vi "Spindexer_Execute.vi"() -> ()   [LabVIEW 2019]
uses:
  Globals/Spindexer_Globals.vi
  <vilib>/Rock Robotics/WPI/ThirdParty/Phoenix-LabVIEW/Motor Controller/Controls/CTRE_Phoenix_MotorControl_ControlMode.ctl
panel:
  in  "Speed control velocity":dbl
  in  "Sensor 5 input":dbl
  in  "Sensor 4 input":dbl
  in  "Sensor 3 input":dbl
  in  "Sensor 2 input":dbl
  in  "Sensor 1 input":dbl
  in  "offset 5":dbl
  in  "Sensor Tolerance 5":dbl
  in  "offset 4":dbl
  in  "Sensor Tolerance 4":dbl
  in  "offset 3":dbl
  in  "Sensor Tolerance 3":dbl
  in  "offset 2":dbl
  in  "Sensor Tolerance 2":dbl
  in  "offset":dbl
  in  "Sensor Tolerance":dbl
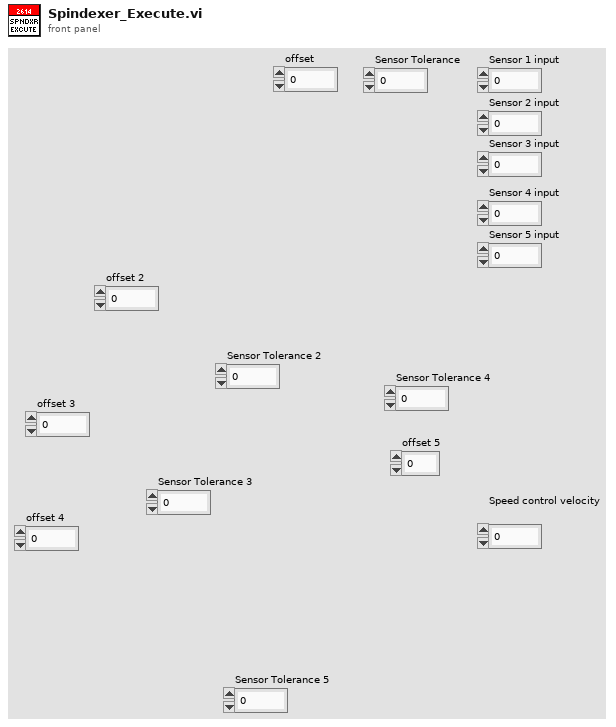
[diagram p1: front panel]
types:
  T1 = typedef "Spindexer_Cluster.ctl" = cluster{"Throttle":dbl, "Fire?":bool, "Intake recently moved?":bool, "Mode":T2, "Sensor in position? ":bool}
  T2 = typedef "Spindexer_mode.ctl" = enum16{"No-Op", "Sensing", "Intaking", "Firing(Speed Control)", "Manual"}
  T3 = typedef "CTRE_Phoenix_MotorControl_ControlMode.ctl" = u16
  T4 = typedef "WPI_MotorControlDeviceRef.ctl" = cluster{"DeviceStatus":errorcluster, "Type":T5, "PWM":cluster{"PWM Channel":T6, "DeadBand":T7}, "CAN":cluster{"Device Number":u8, "SetOutput VI Ref":variant, "GetOutput VI Ref":variant, "Enable VI Ref":variant, "Disable VI Ref":variant, "Data":variant}, "Invert":bool, "DIO PWM":cluster{"PWM \"Enable\" Channel":T6, "DIOChannel":T8, "PWM Rate":dbl}}
  T5 = typedef "WPI_MotorControlType.ctl" = enum16{"PWM", "CAN", "DIO PWM"}
  T6 = typedef "FPGA_DIOPWMChannel.ctl" = enum8{"PWM 0", "PWM 1", "PWM 2", "PWM 3", "PWM 4", "PWM 5", "PWM 6", "PWM 7", "PWM 8", "PWM 9", "PWM MXP 0", "PWM MXP 1", "PWM MXP 2", "PWM MXP 3", "PWM MXP 4", "PWM MXP 5", "PWM MXP 6", "PWM MXP 7", "PWM MXP 8", "PWM MXP 9", "Invalid"}
  T7 = typedef "WPI_PWMDeadband.ctl" = cluster{"Name":string, "maxPositivePwm":i32, "minPositivePwm":i32, "centerPwm":i32, "maxNegativePwm":i32, "minNegativePwm":i32, "angularRange":u16}
  T8 = typedef "FPGA_DIOChannel.ctl" = enum8{"DIO 0", "DIO 1", "DIO 2", "DIO 3", "DIO 4", "DIO 5", "DIO 6", "DIO 7", "DIO 8", "DIO 9", "DIO MXP 0", "DIO MXP 1", "DIO MXP 2", "DIO MXP 3", "DIO MXP 4", "DIO MXP 5", "DIO MXP 6", "DIO MXP 7", "DIO MXP 8", "DIO MXP 9", "DIO MXP 10", "DIO MXP 11", "DIO MXP 12", "DIO MXP 13", "DIO MXP 14", "DIO MXP 15", "SPI Port CS1", "SPI Port CS2", "SPI Port CS3", "SPI Port MISO", "SPI Port MOSI", "Invalid"}
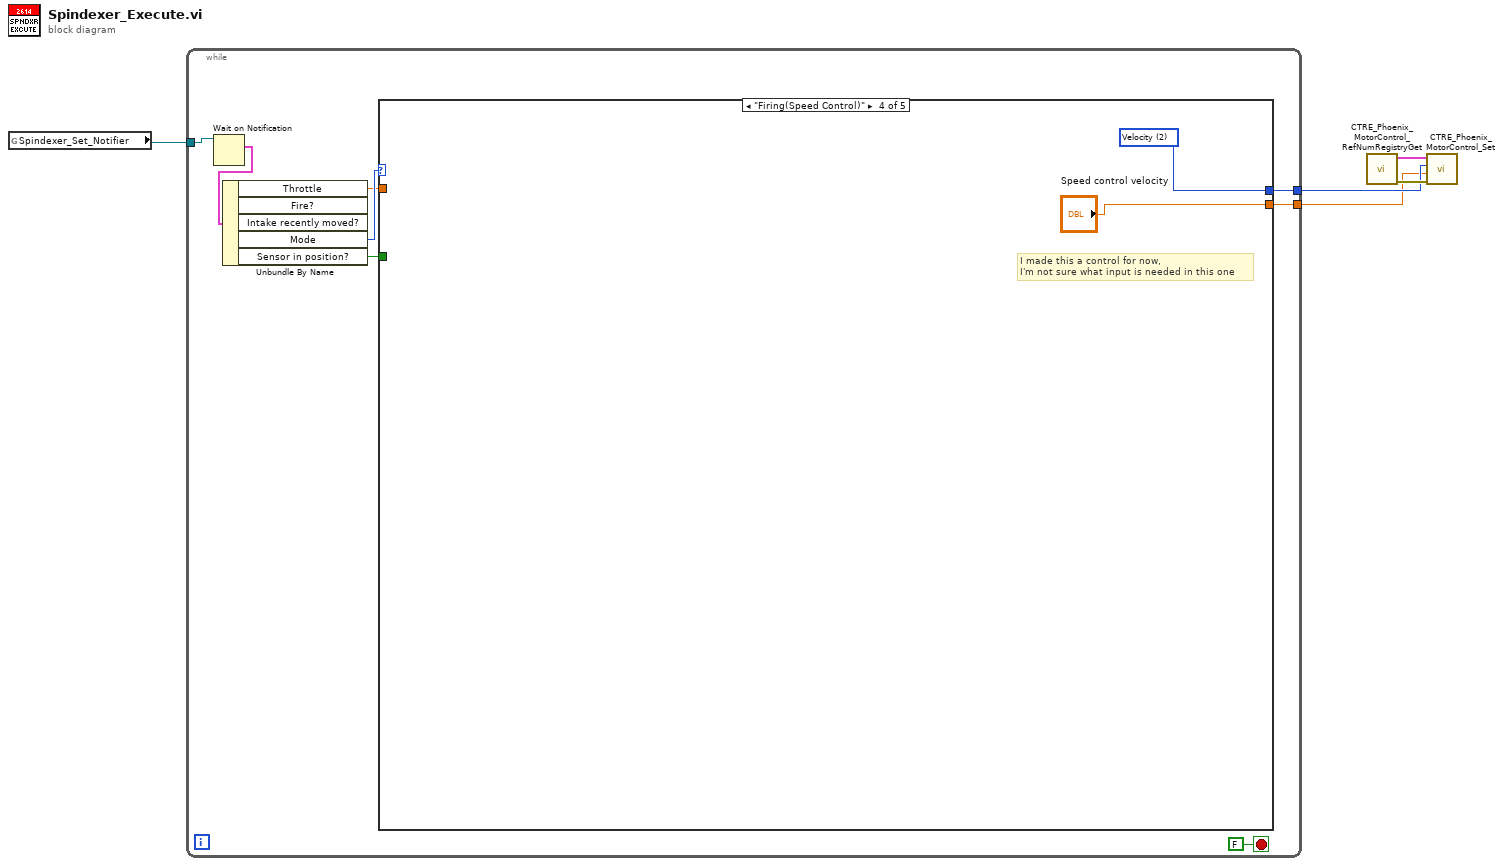
[diagram p0: block diagram]
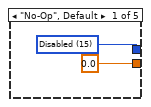
[diagram p2: hidden frame]
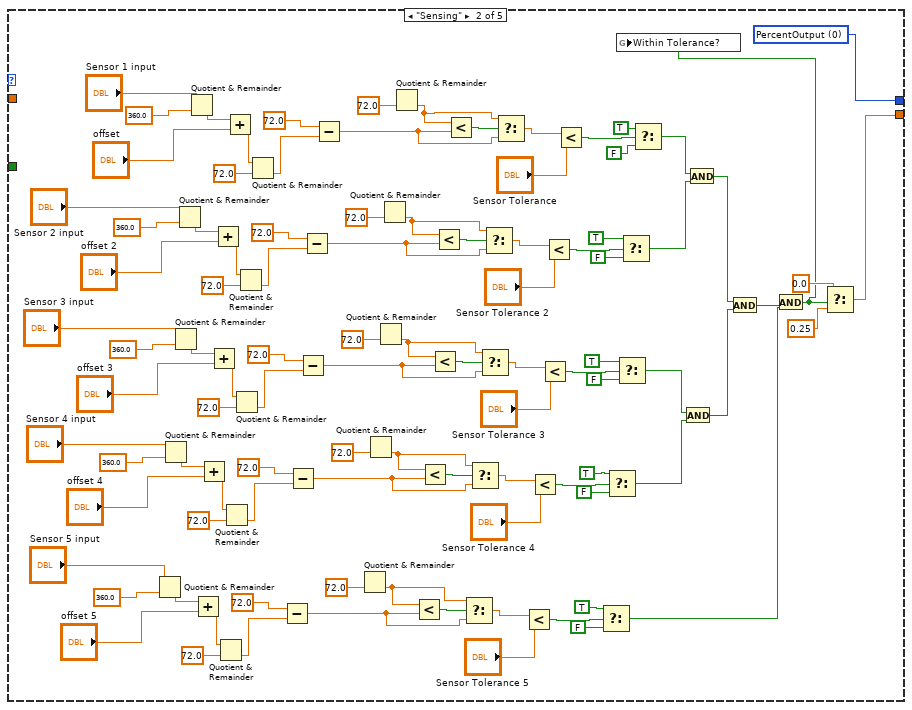
[diagram p3: hidden frame]
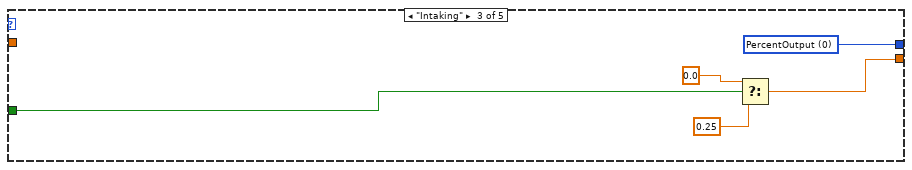
[diagram p4: hidden frame]
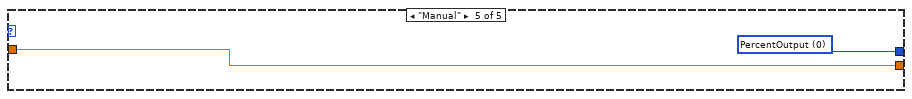
[diagram p5: hidden frame]
diagram:
  n1 = global read "Spindexer_Globals.vi" "Spindexer_Set_Notifier"() -> (w5:refnum<notifier>)
  n2 = while {
    tunnel: w5 -> [w12]
    tunnel: [w9] -> w2
    tunnel: [w7] -> w1
    stop <- FALSE stop-if-true
    n3 = Wait on Notification(notifier=w12) -> (notification=w11:T1)  [unwired: 3 in, 3 out]
    n4 = Unbundle By Name(w11) -> ("Throttle"=w8:dbl, "Mode"=w10:T2, "Sensor in position?"=w6:bool)  [unwired: 2 out]
    n5 = case shown="\"Firing(Speed Control)\"" w10 {
      tunnel: [w14 w113 w118 w120 w121] -> w9
      tunnel: w8 -> [_ _ _ _ w122]
      tunnel: [0.0 ("Throttle") w17 w114 "Speed control velocity" w122] -> w7
      tunnel: w6 -> [_ _ w117 _ _]
      frame "No-Op", Default {
        w14 = T3 15 items=["PercentOutput"=0, "Position"=1, "Velocity"=2, "Current"=3, "Follower"=5, "MotionProfile"=6, "MotionMagic"=7, "MotionProfileArc"=10, "Disabled"=15] ("Control Mode")
      }
      frame "Sensing" {
        w113 = T3 0 items=["PercentOutput"=0, "Position"=1, "Velocity"=2, "Current"=3, "Follower"=5, "MotionProfile"=6, "MotionMagic"=7, "MotionProfileArc"=10, "Disabled"=15] ("Control Mode")
        n6 = Quotient & Remainder(x="Sensor 5 input", y=360.0) -> (floor(x/y)=w53:dbl)  [unwired: 1 out]
        n7 = Quotient & Remainder(x="Sensor 4 input", y=360.0) -> (floor(x/y)=w65:dbl)  [unwired: 1 out]
        n8 = Quotient & Remainder(x="Sensor 3 input", y=360.0) -> (floor(x/y)=w77:dbl)  [unwired: 1 out]
        n9 = Quotient & Remainder(x="Sensor 2 input", y=360.0) -> (floor(x/y)=w89:dbl)  [unwired: 1 out]
        n10 = Quotient & Remainder(x="Sensor 1 input", y=360.0) -> (floor(x/y)=w101:dbl)  [unwired: 1 out]
        n11 = Add(x=w53, y="offset 5") -> (x+y=w52:dbl)
        n12 = Add(x=w65, y="offset 4") -> (x+y=w64:dbl)
        n13 = Add(x=w77, y="offset 3") -> (x+y=w76:dbl)
        n14 = Add(x=w89, y="offset 2") -> (x+y=w88:dbl)
        n15 = Quotient & Remainder(x=w52, y=72.0) -> (floor(x/y)=w61:dbl)  [unwired: 1 out]
        n16 = Quotient & Remainder(x=w64, y=72.0) -> (floor(x/y)=w73:dbl)  [unwired: 1 out]
        n17 = Add(x=w101, y="offset") -> (x+y=w100:dbl)
        n18 = Quotient & Remainder(x=w76, y=72.0) -> (floor(x/y)=w85:dbl)  [unwired: 1 out]
        n19 = Quotient & Remainder(x=w88, y=72.0) -> (floor(x/y)=w97:dbl)  [unwired: 1 out]
        n20 = Quotient & Remainder(x=w100, y=72.0) -> (floor(x/y)=w111:dbl)  [unwired: 1 out]
        n21 = Subtract(x=72.0, y=w61) -> (x-y=w58:dbl)
        n22 = Subtract(x=72.0, y=w73) -> (x-y=w70:dbl)
        n23 = Subtract(x=72.0, y=w85) -> (x-y=w82:dbl)
        n24 = Subtract(x=72.0, y=w97) -> (x-y=w94:dbl)
        n25 = Subtract(x=72.0, y=w111) -> (x-y=w106:dbl)
        n26 = Quotient & Remainder(y=72.0) -> (floor(x/y)=w50:dbl)  [unwired: 1 in, 1 out]
        n27 = Quotient & Remainder(y=72.0) -> (floor(x/y)=w45:dbl)  [unwired: 1 in, 1 out]
        n28 = Quotient & Remainder(y=72.0) -> (floor(x/y)=w44:dbl)  [unwired: 1 in, 1 out]
        n29 = Quotient & Remainder(y=72.0) -> (floor(x/y)=w43:dbl)  [unwired: 1 in, 1 out]
        n30 = Quotient & Remainder(y=72.0) -> (floor(x/y)=w107:dbl)  [unwired: 1 in, 1 out]
        n31 = Less?(x=w50, y=w58) -> (x < y?=w59:bool)
        n32 = Less?(x=w45, y=w70) -> (x < y?=w71:bool)
        n33 = Less?(x=w44, y=w82) -> (x < y?=w83:bool)
        n34 = Less?(x=w43, y=w94) -> (x < y?=w95:bool)
        n35 = Less?(x=w107, y=w106) -> (x < y?=w109:bool)
        n36 = Select(t=w50, s=w59, f=w58) -> (s? t:f=w57:dbl)
        n37 = Select(t=w45, s=w71, f=w70) -> (s? t:f=w69:dbl)
        n38 = Select(t=w44, s=w83, f=w82) -> (s? t:f=w81:dbl)
        n39 = Select(t=w43, s=w95, f=w94) -> (s? t:f=w93:dbl)
        n40 = Select(t=w107, s=w109, f=w106) -> (s? t:f=w105:dbl)
        n41 = Less?(x=w57, y="Sensor Tolerance 5") -> (x < y?=w55:bool)
        n42 = Less?(x=w69, y="Sensor Tolerance 4") -> (x < y?=w67:bool)
        n43 = Less?(x=w81, y="Sensor Tolerance 3") -> (x < y?=w79:bool)
        n44 = Less?(x=w93, y="Sensor Tolerance 2") -> (x < y?=w91:bool)
        n45 = Less?(x=w105, y="Sensor Tolerance") -> (x < y?=w103:bool)
        n46 = Select(t=TRUE, s=w55, f=FALSE) -> (s? t:f=w20:bool)
        n47 = Select(t=TRUE, s=w67, f=FALSE) -> (s? t:f=w24:bool)
        n48 = Select(t=TRUE, s=w79, f=FALSE) -> (s? t:f=w25:bool)
        n49 = Select(t=TRUE, s=w91, f=FALSE) -> (s? t:f=w26:bool)
        n50 = Select(t=TRUE, s=w103, f=FALSE) -> (s? t:f=w27:bool)
        n51 = And(x=w25, y=w24) -> (x .and. y?=w22:bool)
        n52 = And(x=w27, y=w26) -> (x .and. y?=w23:bool)
        n53 = And(x=w23, y=w22) -> (x .and. y?=w21:bool)
        n54 = And(x=w21, y=w20) -> (x .and. y?=w16:bool)
        n55 = global write "Spindexer_Globals.vi" "Within Tolerance?"(w16) -> ()
        n56 = Select(t=0.0, s=w16, f=0.25) -> (s? t:f=w17:dbl)
      }
      frame "Intaking" {
        w118 = T3 0 items=["PercentOutput"=0, "Position"=1, "Velocity"=2, "Current"=3, "Follower"=5, "MotionProfile"=6, "MotionMagic"=7, "MotionProfileArc"=10, "Disabled"=15] ("Control Mode")
        n57 = Select(t=0.0, s=w117, f=0.25) -> (s? t:f=w114:dbl)
      }
      frame "Firing(Speed Control)" {
        w120 = T3 2 items=["PercentOutput"=0, "Position"=1, "Velocity"=2, "Current"=3, "Follower"=5, "MotionProfile"=6, "MotionMagic"=7, "MotionProfileArc"=10, "Disabled"=15] ("Control Mode")
        # "I made this a control for now, \nI'm not sure what input is needed in this one"
      }
      frame "Manual" {
        w121 = T3 0 items=["PercentOutput"=0, "Position"=1, "Velocity"=2, "Current"=3, "Follower"=5, "MotionProfile"=6, "MotionMagic"=7, "MotionProfileArc"=10, "Disabled"=15] ("Control Mode")
      }
    }
  }
  n58 = call <vilib>:"CTRE_Phoenix_MotorControl_RefNumRegistryGet.vi"() -> ("error out"=w4:errorcluster, "PhoenixMotorControlDevRef"=w3:T4)  [unwired: 10 in]
  n59 = call <vilib>:"CTRE_Phoenix_MotorControl_Set.vi"("error in (no error)"=w4, "Output"=w1, "Control Mode"=w2, "PhoenixMotorControlDevRef"=w3) -> ()  [unwired: 6 in, 2 out]
